vi "Setup_3D_Earth.vi"() -> (0 "error out":errorcluster, 3 "SceneObject out":refnum<vi>)   [LabVIEW 2014]
uses:
  <vilib>/picture/3D Picture Control/Object/Create Object (name).vi
  <vilib>/picture/3D Picture Control/NI_3D Picture Control.lvlib
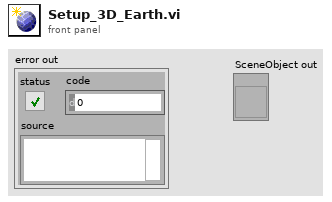
[diagram p1: front panel]
types:
  T1 = enum16{"As a Decal", "With Modulation", "With Blending", "As a replacement"}
  T2 = typedef "imagedata.ctl" = cluster{"image type":i32, "image depth":i32, "image":u8[], "mask":u8[], "colors":u32[], "Rectangle":cluster{"left":i16, "top":i16, "right":i16, "bottom":i16}}
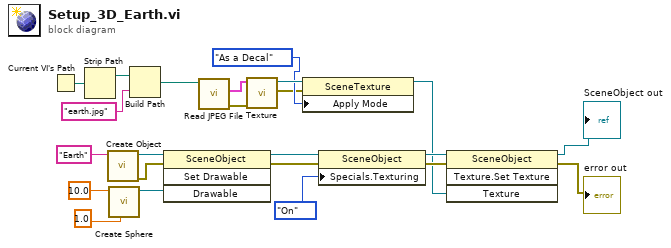
[diagram p0: block diagram]
diagram:
  n1 = Current VI's Path() -> (path=w10:path)
  n2 = Strip Path(path=w10) -> (stripped path=w14:path)  [unwired: 1 out]
  n3 = call-poly <vilib>:"Create Object.vi"("Name"="Earth") -> ("error out"=w8:errorcluster, "Scene:New Object"=w6:refnum<vi>)  [unwired: 9 in]
  n4 = call <vilib>:"Create Sphere.vi"("Detail"=sgl 1.0, "Radius"=sgl 10.0) -> ("New Sphere Refnum"=w7:refnum<vi>)  [unwired: 1 in, 8 out]
  n5 = Build Path(base path=w14, name or relative path="earth.jpg" ("Name")) -> (appended path=w11:path)
  n6 = invoke class="SceneObject" method="Set Drawable"(reference=w6, error in=w8, "Drawable"=w7) -> (reference out=w20:refnum<vi>, error out=w21:errorcluster)  [unwired: 1 in, 2 out]
  n7 = call <vilib>:"Read JPEG File.vi"("path to JPEG file"=w11) -> ("error out"=w2:errorcluster, "image data"=w17:T2)  [unwired: 1 in, 8 out]
  n8 = call <vilib>:"Texture.vi"("error in (no error)"=w2, "Image"=w17) -> ("error out"=w3:errorcluster, "New Texture Refnum"=w18:refnum<vi>)  [unwired: 8 out]
  n9 = property class="SceneTexture"(reference=w18, error in=w3, "Apply Mode"=T1."As a Decal") -> (reference out=w13:refnum<vi>)  [unwired: 1 out]
  n10 = property class="SceneObject"(reference=w20, error in=w21, "Specials.Texturing"=enum16{"Inherit Value", "Off", "On"}."On" ("Specials:Texturing")) -> (reference out=w22:refnum<vi>, error out=w23:errorcluster)
  n11 = invoke class="SceneObject" method="Texture.Set Texture"(reference=w22, error in=w23, "Texture"=w13) -> (reference out=→"SceneObject out":refnum<vi>, error out=→"error out":errorcluster)  [unwired: 1 in, 2 out]
